vi "(SubVI) organize theme compare.vi"(1 "Talent array":string[](array[string]), 2 "Theme compare":string[][](array[string])) -> (0 "organize theme compare":string[][](array[string]))   [LabVIEW 2022 SP3]
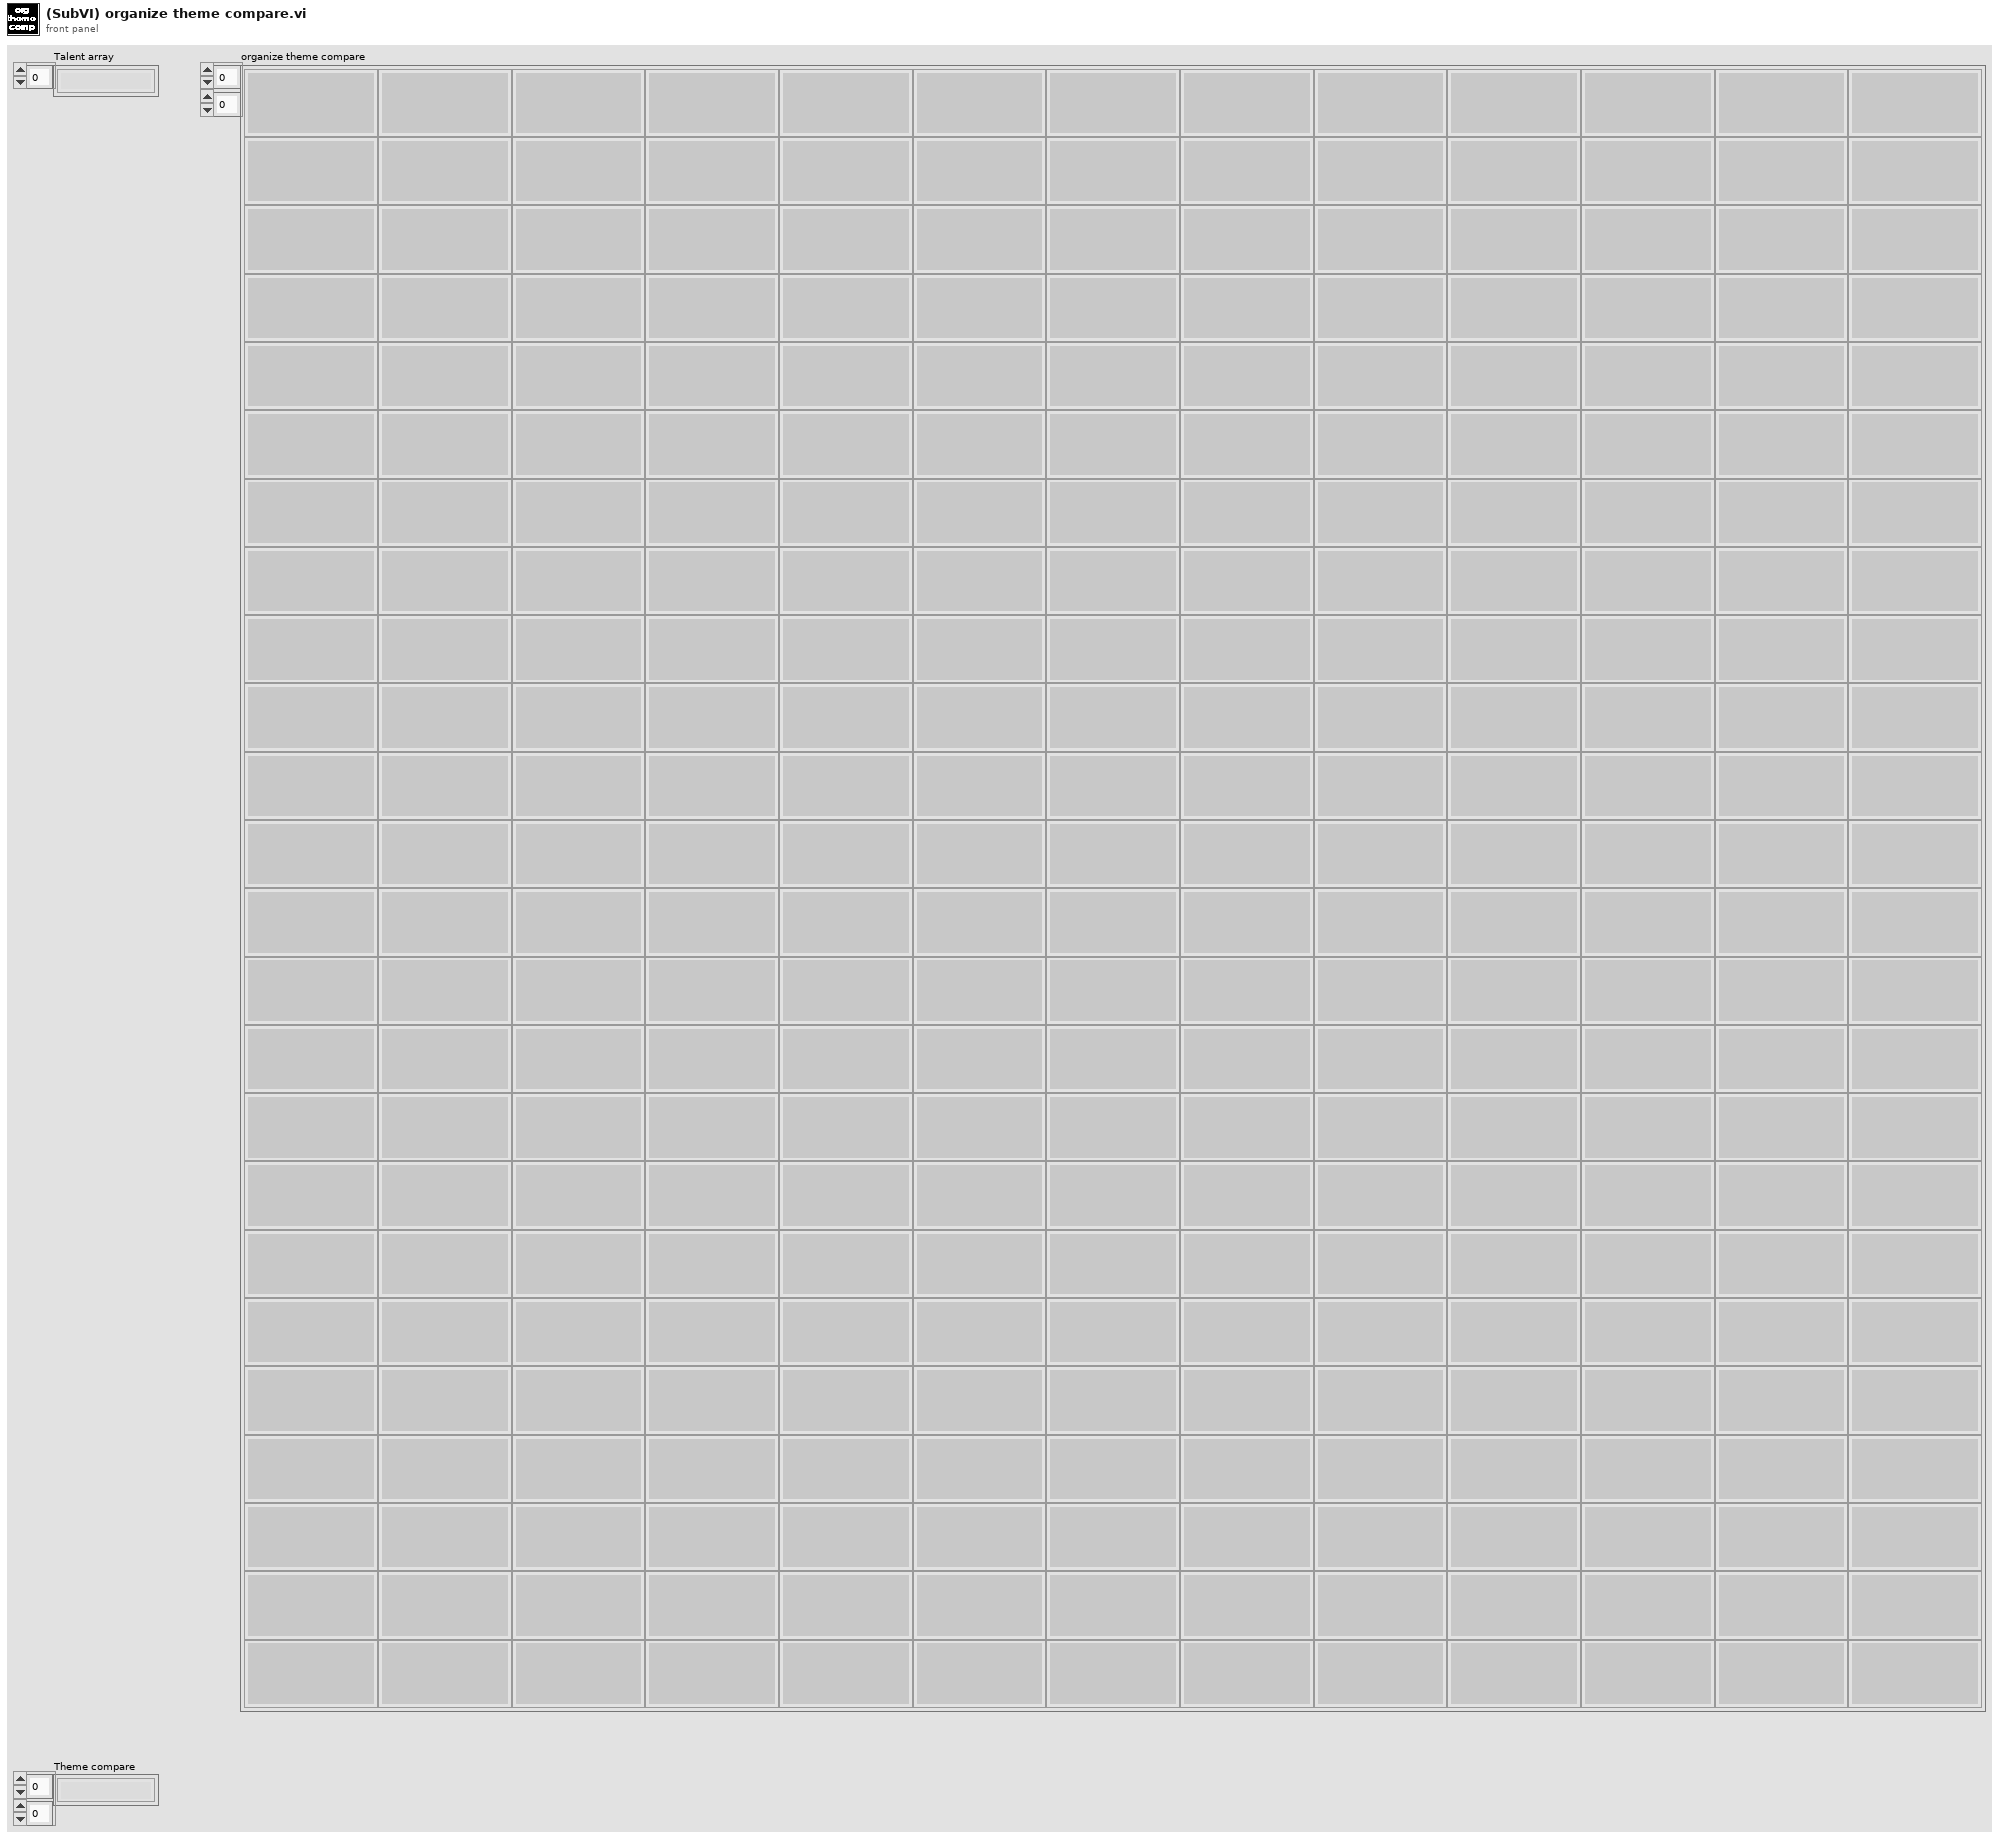
[diagram p1: front panel]
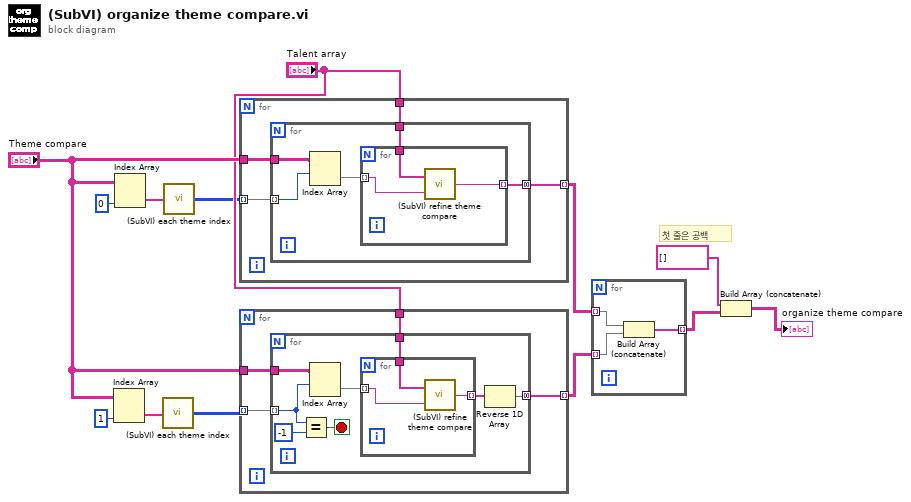
[diagram p0: block diagram]
diagram:
  # "첫 줄은 공백"
  n1 = Index Array(array="Theme compare", index (col)=1 ("disabled index (col)")) -> (element=w7:string[])  [unwired: 1 in]
  n2 = Index Array(array="Theme compare", index (col)=0 ("disabled index (col)")) -> (element=w6:string[])  [unwired: 1 in]
  n3 = call "(SubVI) each theme index.vi"("Theme compare"=w7) -> ("theme index"=w10:i32[][])
  n4 = call "(SubVI) each theme index.vi"("Theme compare"=w6) -> ("theme index"=w8:i32[][])
  n5 = for {
    tunnel: w8 -> [w17] mode=indexing
    tunnel: "Theme compare" -> [w16]
    tunnel: "Talent array" -> [w15]
    tunnel: [w14] -> w12 mode=indexing
    n6 = for {
      tunnel: w17 -> [w21] mode=indexing
      tunnel: w16 -> [w22]
      tunnel: w15 -> [w19]
      tunnel: [w18] -> w14 mode=concatenating
      n7 = Index Array(array=w22, index (row)=w21) -> (element=w20:string[])  [unwired: 1 in]
      n8 = for {
        tunnel: w20 -> [w24] mode=indexing
        tunnel: w19 -> [w25]
        tunnel: [w23] -> w18 mode=indexing
        n9 = call "(SubVI) refine theme compare.vi"("String in"=w24, "Talent array"=w25) -> ("refine theme compare"=w23:string)
      }
    }
  }
  n10 = for {
    tunnel: w10 -> [w29] mode=indexing
    tunnel: "Theme compare" -> [w28]
    tunnel: "Talent array" -> [w27]
    tunnel: [w26] -> w13 mode=indexing
    n11 = for {
      tunnel: w29 -> [w31] mode=indexing
      tunnel: w28 -> [w37]
      tunnel: w27 -> [w35]
      tunnel: [w34] -> w26 mode=concatenating
      stop <- w32 stop-if-true
      n12 = Equal?(x=w31, y=-1) -> (x = y?=w32:bool)
      n13 = Index Array(array=w37, index (row)=w31) -> (element=w36:string[])  [unwired: 1 in]
      n14 = for {
        tunnel: w36 -> [w39] mode=indexing
        tunnel: w35 -> [w40]
        tunnel: [w38] -> w33 mode=indexing
        n15 = call "(SubVI) refine theme compare.vi"("String in"=w39, "Talent array"=w40) -> ("refine theme compare"=w38:string)
      }
      n16 = Reverse 1D Array(array=w33) -> (reversed array=w34:string[])
    }
  }
  n17 = for {
    tunnel: w12 -> [w43] mode=indexing
    tunnel: w13 -> [w42] mode=indexing
    tunnel: [w41] -> w3 mode=indexing
    n18 = Build Array (concatenate)(w43, w42) -> (w41:string[])
  }
  n19 = Build Array (concatenate)(string[] [], w3) -> (→"organize theme compare":string[][])
